vi "class_load_single_image.vi"(11 "Path":path) -> (3 "Image":T1(plugin-control))   [LabVIEW 2017]
uses:
  data_loder/data_loader_single_image/data_loader_single_image.lvclass
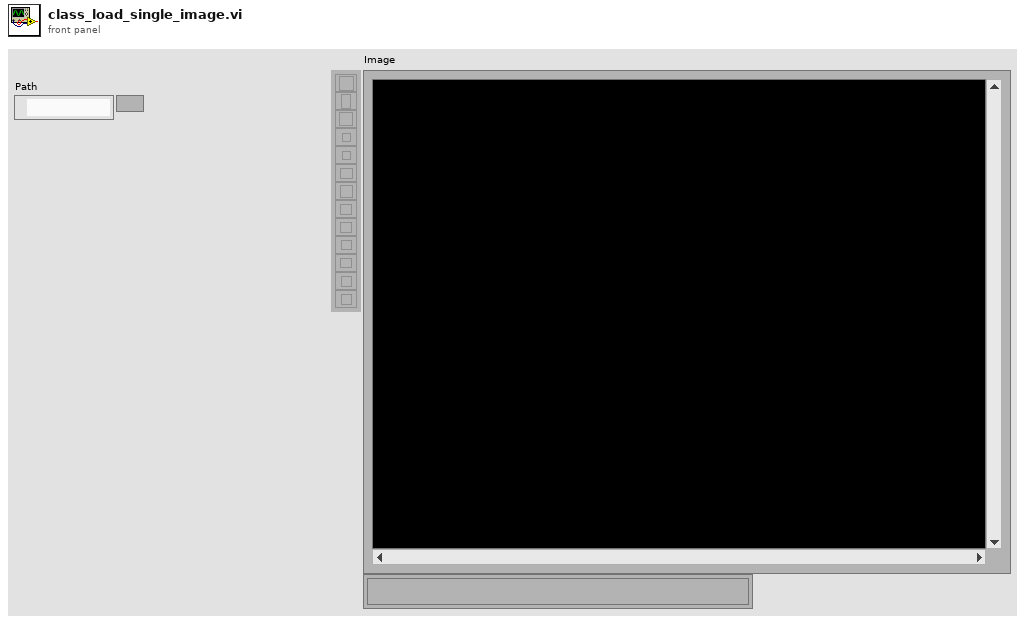
[diagram p1: front panel]
types:
  T1 = typedef "IMAQ Image.ctl" = refnum<image>
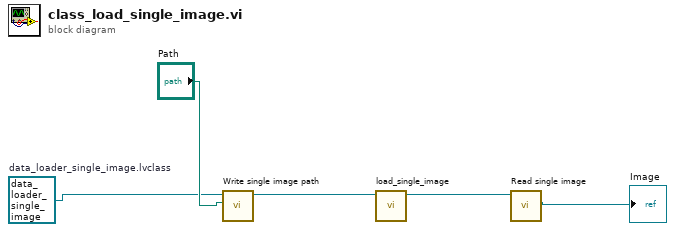
[diagram p0: block diagram]
diagram:
  w2 = refnum<class "data_loader_single_image.lvclass"> refnum  # data_loader_single_image.lvclass
  n1 = call-dynamic "Write single image path.vi"("image path"="Path", "data_loder_single_image in"=w2) -> ("data_loder_single_image out"=w5:refnum<class "data_loader_single_image.lvclass">)  [unwired: 8 in, 1 out]
  n2 = call-dynamic "load_single_image.vi"("data_loader_single_image in"=w5) -> ("data_loader_single_image out"=w4:refnum<class "data_loader_single_image.lvclass">)  [unwired: 9 in, 1 out]
  n3 = call-dynamic "Read single image.vi"("data_loder_single_image in"=w4) -> ("Image"=→"Image":T1)  [unwired: 8 in, 2 out]
